vi "_Destroy.vi"(8 "error in (no error)":errorcluster, 11 "Stepper in":refnum<class "Stepper.lvclass">) -> (0 "error out":errorcluster)   [LabVIEW 2017, in "Stepper.lvclass"]
uses:
  Stepper.lvclass
  Stepper.lvclass/Stepper.ctl
  <vilib>/Utility/config.llb/Write Key (Double).vi
  Utility Classes/Scannable/Scannable.lvclass
  <vilib>/Utility/config.llb/NI_LVConfig.lvlib
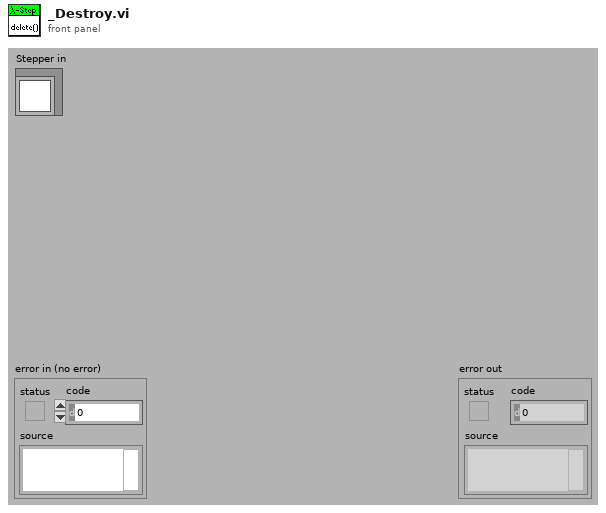
[diagram p1: front panel]
types:
  T1 = typedef "NI_LVConfig.lvlib/Config Data RefNum.ctl" = refnum<k1>
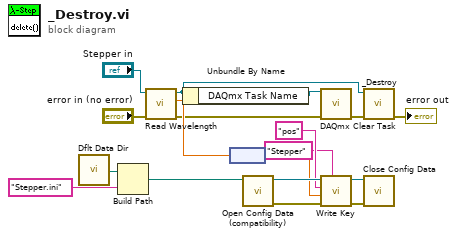
[diagram p0: block diagram]
diagram:
  n1 = call <vilib>:"Dflt Data Dir.vi"() -> ("App:Default Data Directory"=w14:path)
  n2 = Build Path(base path=w14, name or relative path="Stepper.ini") -> (appended path=w12:path)
  n3 = call-dynamic "Read Wavelength.vi"("error in (no error)"="error in (no error)", "Stepper.lvclass in"="Stepper in") -> ("error out"=w2:errorcluster, "Current Wavelength"=w5:dbl[unit], "Stepper.lvclass out"=w6:refnum<class "Stepper.lvclass">)  [unwired: 7 out]
  n4 = Unbundle By Name(w6) -> ("DAQmx Task Name"=w16:refnum<k21>)
  n5 = node(w5) -> (w4:dbl)
  n6 = call <vilib>:"Open Config Data (compatibility).vi"("configuration file path"=w12) -> ("error out"=w10:errorcluster, "refnum"=w11:T1)  [unwired: 8 in, 1 out]
  n7 = call <vilib>:"DAQmx Clear Task.vi"("task in"=w16, "error in"=w2) -> ("error out"=w15:errorcluster)  [unwired: 13 out]
  n8 = call-poly <vilib>:"Write Key.vi"("section"="Stepper", "error in (no error)"=w10, "value"=w4, "key"="pos", "refnum"=w11) -> ("error out"=w7:errorcluster, "refnum out"=w8:T1)  [unwired: 3 in, 2 out]
  n9 = call-parent "_Destroy.vi"("error in (no error)"=w15, "Instrument in"=w6) -> ("error out"=→"error out":errorcluster)  [unwired: 9 out]
  n10 = call <vilib>:"Close Config Data.vi"("error in (no error)"=w7, "refnum"=w8) -> ()  [unwired: 1 in, 9 out]
